vi "Align cRIO Programming Mode.vi"(5 "Password":string, 7 "User Name":string, 8 "error in (no error)":errorcluster, 10 "Slots Configuration":T1[](array[typedef]), 11 "Target (localhost)":refnum<k21>="localhost") -> (0 "error out":errorcluster)   [LabVIEW 2020, in "SEECD System Explorer.lvlib"]
doc: "Based on FPGAScanInterfaceMode input, this VI aligns actual Slot Programming Mode:\n- FPGAScanInterfaceMode = 0 (Use Current), we do nothing. We don't even check current settings (because, it's super slow (SystemConfiguration API)).\n- FPGAScanInterfaceMode = 1 (FPGA) or (Scan mode), we retrieves Product Name and if it's a ni-rio product, checks agains Input list whether it supports the Slot Programming Mode. Then, for detected Slots, we ensure the Slot Programming Mode value is aligned to FPGAScanInterfaceMode and change it if required."
uses:
  SEECD System Explorer.lvlib
  Type Defs/Slot Programming Mode.ctl
  <vilib>/nisyscfg/Filter Mode.ctl
  <vilib>/nisyscfg/Save Changes (Hardware).vi
  <vilib>/nisyscfg/Close (Hardware).vi
  <vilib>/nisyscfg/Close (Filter).vi
  <vilib>/nisyscfg/Close (System).vi
  <vilib>/nisyscfg/nisyscfg.lvlib
  <resource>/objmgr/nisysapi.rc
  <resource>/objmgr/nicontrollersysapi.rc
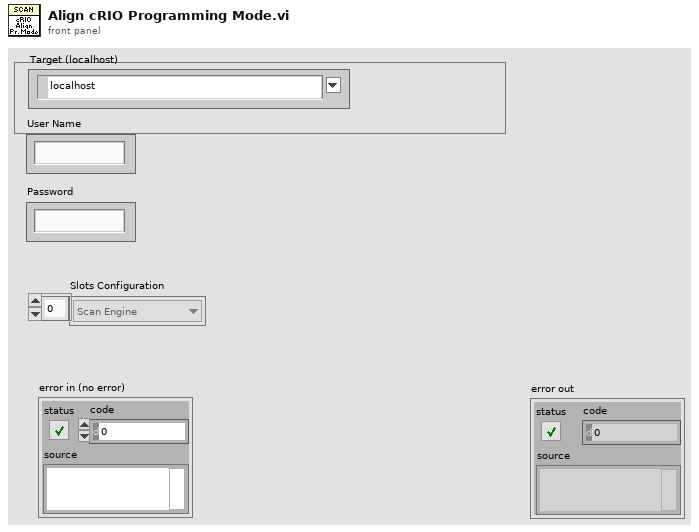
[diagram p1: front panel]
types:
  T1 = typedef "SEECD System Explorer.lvlib/Slot Programming Mode.ctl" = enum16{"Don't Modify", "Scan Engine", "LabVIEW FPGA", "NI-DAQmx"}
  T2 = typedef "nisyscfg.lvlib/Filter Mode.ctl" = i32
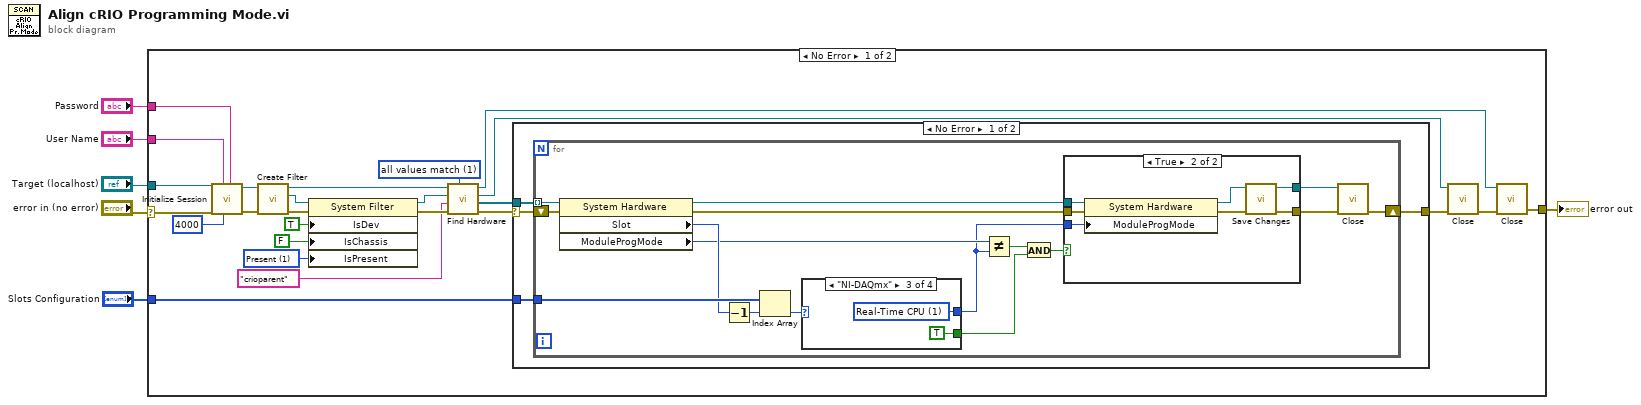
[diagram p0: block diagram]
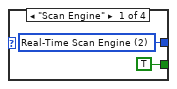
[diagram p3: hidden frame]
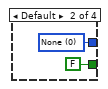
[diagram p4: hidden frame]
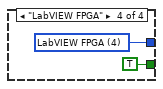
[diagram p5: hidden frame]
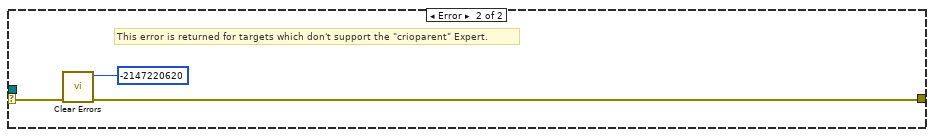
[diagram p6: hidden frame]
diagram:
  n1 = case shown="No Error" "error in (no error)" {
    selector: "error in (no error)" -> [w27 w72]
    tunnel: "Target (localhost)" -> [w31 _]
    tunnel: "User Name" -> [w30 _]
    tunnel: "Password" -> [w29 _]
    tunnel: [w28 w72] -> w3
    tunnel: "Slots Configuration" -> [w7 _]
    frame No Error {
      w10 = 1 items=["Initializing"=-2, "Unknown"=-1, "Not Present"=0, "Present"=1] ("Devices & Chassis:Is Present")
      w17 = T2 1 items=["all values match"=1, "any value matches"=2, "values do not match"=3, "all properties exist"=4] ("filter mode (all values match)")
      n2 = call <vilib>:"Initialize Session.vi"("Password"=w29, "Connect Timeout (4000 ms)"=u32 4000, "User Name"=w30, "error in (no error)"=w27, "Target (localhost)"=w31) -> ("error out"=w19:errorcluster, "Session out"=w22:refnum<k21>)  [unwired: 5 in]
      n3 = call <vilib>:"Create Filter.vi"("error in (no error)"=w19, "Session in"=w22) -> ("error out"=w24:errorcluster, "Filter out"=w23:refnum<k20>, "Session out"=w21:refnum<k21>)  [unwired: 7 in]
      n4 = property class="System Filter"(reference=w23, error in=w24, "IsDev"=TRUE ("Is Device"), "IsChassis"=FALSE ("Is Chassis"), "IsPresent"=w10) -> (reference out=w18:refnum<k20>, error out=w20:errorcluster)
      n5 = call <vilib>:"Find Hardware.vi"("Filter Mode (all values match)"=w17, "error in (no error)"=w20, "Experts"="crioparent" ("Expert Info:Expert Name"), "Filter in"=w18, "Session in"=w21) -> ("error out"=w8:errorcluster, "Resources out"=w26:refnum<k20>[], "Filter out"=w15:refnum<k20>, "Session out"=w25:refnum<k21>)  [unwired: 3 out]
      n6 = case shown="No Error" w8 {
        selector: w8 -> [w33 w71]
        tunnel: w26 -> [w35 _]
        tunnel: [w34 w69] -> w14
        tunnel: w7 -> [w32 _]
        frame No Error {
          n7 = for {
            tunnel: w35 -> [w50] mode=indexing
            shift-right: [w51] -> w34
            shift-left: w33 -> [w49]
            tunnel: w32 -> [w48]
            n8 = property class="System Hardware"(reference=w50, error in=w49) -> (reference out=w42:refnum<k20>, error out=w41:errorcluster, "Slot"=w46:i32, "ModuleProgMode"=w40:u32)
            n9 = Decrement(x=w46) -> (x-1=w47:i32)
            n10 = Index Array(array=w48, index=w47) -> (element=w45:T1)
            n11 = case shown="\"NI-DAQmx\"" w45 {
              tunnel: [w62 w64 w66 w68] -> w36
              tunnel: [TRUE FALSE TRUE TRUE] -> w37
              frame "Scan Engine" {
                w62 = u32 2 items=["None"=0, "Real-Time CPU"=1, "Real-Time Scan Engine"=2, "LabVIEW FPGA"=4] ("Devices & Chassis:Bus Specific:cRIO Module Programming Mode")
              }
              frame Default {
                w64 = u32 0 items=["None"=0, "Real-Time CPU"=1, "Real-Time Scan Engine"=2, "LabVIEW FPGA"=4] ("Devices & Chassis:Bus Specific:cRIO Module Programming Mode")
              }
              frame "NI-DAQmx" {
                w66 = u32 1 items=["None"=0, "Real-Time CPU"=1, "Real-Time Scan Engine"=2, "LabVIEW FPGA"=4] ("Devices & Chassis:Bus Specific:cRIO Module Programming Mode")
              }
              frame "LabVIEW FPGA" {
                w68 = u32 4 items=["None"=0, "Real-Time CPU"=1, "Real-Time Scan Engine"=2, "LabVIEW FPGA"=4] ("Devices & Chassis:Bus Specific:cRIO Module Programming Mode")
              }
            }
            n12 = Not Equal?(x=w40, y=w36) -> (x != y?=w39:bool)
            n13 = And(x=w39, y=w37) -> (x .and. y?=w38:bool)
            n14 = case shown="True" w38 {
              tunnel: w42 -> [w53 w60]
              tunnel: w41 -> [w52 w59]
              tunnel: [w53 w55] -> w44
              tunnel: [w52 w56] -> w43
              tunnel: w36 -> [_ w54]
              frame False {
                # "Already set with right Pr. mode.\nor absent."
              }
              frame True {
                n15 = property class="System Hardware"(reference=w60, error in=w59, "ModuleProgMode"=w54) -> (reference out=w57:refnum<k20>, error out=w58:errorcluster)
                n16 = call-poly <vilib>:"Save Changes.vi"("error in (no error)"=w58, "Resource in"=w57) -> ("error out"=w56:errorcluster, "Resource out"=w55:refnum<k20>)  [unwired: 6 in, 2 out]
              }
            }
            n17 = call-poly <vilib>:"Close.vi"("error in (no error)"=w43, "Resource in"=w44) -> ("error out"=w51:errorcluster)  [unwired: 9 in]
          }
        }
        frame Error {
          # "This error is returned for targets which don't support the \"crioparent\" Expert."
          n18 = call <vilib>:"Clear Errors.vi"("error in (no error)"=w71, "specific error code to clear (0: all)"=-2147220620) -> ("error out"=w69:errorcluster)  [unwired: 4 in, 1 out]
        }
      }
      n19 = call-poly <vilib>:"Close.vi"("error in (no error)"=w14, "Filter in"=w15) -> ("error out"=w16:errorcluster)  [unwired: 9 in]
      n20 = call-poly <vilib>:"Close.vi"("error in (no error)"=w16, "Session in"=w25) -> ("error out"=w28:errorcluster)  [unwired: 9 in]
    }
    frame Error {
    }
  }
  "error out" <- w3
